vi "sub_MEMS Value to Frequency.vi"(11 "MEMS FAST":dbl(slide) caption="Fast" scale=0.0..300000.0) -> (3 "Ticks":u32)   [LabVIEW 2015]
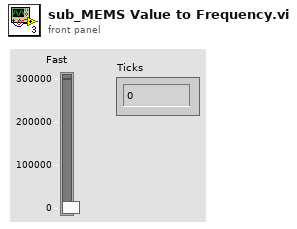
[diagram p1: front panel]
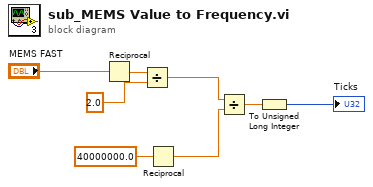
[diagram p0: block diagram]
diagram:
  n1 = Reciprocal(x="MEMS FAST") -> (1/x=w7:dbl)
  n2 = Divide(x=w7, y=2.0) -> (x/y=w5:dbl)
  n3 = Reciprocal(x=40000000.0) -> (1/x=w4:dbl)
  n4 = Divide(x=w5, y=w4) -> (x/y=w2:dbl)
  n5 = To Unsigned Long Integer(number=w2) -> (unsigned 32bit integer=→"Ticks":u32)
